vi "CliListBlocks.vi"(0 "ref in":u64, 11 "error in (no error)":errorcluster) -> (4 "ref out":u64, 6 "Result":i32, 8 "BlockList":T1, 15 "error out":errorcluster)   [LabVIEW 2019, in "Snap7.lvlib"]
uses:
  Snap7.lvlib
  windows/lv_snap7.dll
panel:
  in  "var BlockList":T1
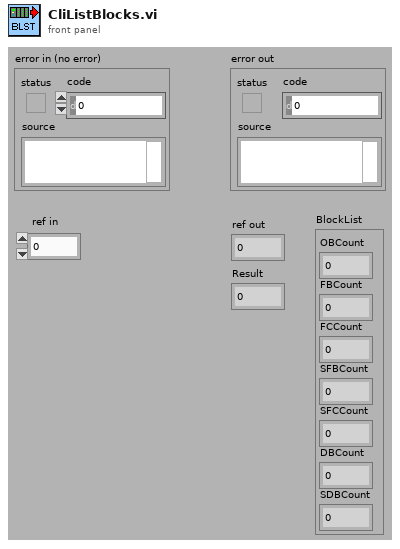
[diagram p1: front panel]
types:
  T1 = cluster{"OBCount":i32, "FBCount":i32, "FCCount":i32, "SFBCount":i32, "SFCCount":i32, "DBCount":i32, "SDBCount":i32}
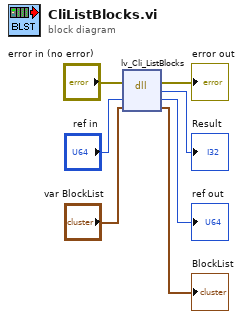
[diagram p0: block diagram]
diagram:
  n1 = dll-call lib="PTH2Xabs DSVNHLCEPStrunk性能试验台SourcesSnap7libwindowslv_snap7.dll" fn="lv_Cli_ListBlocks"(error in="error in (no error)", "Client"="ref in", "Cluster"="var BlockList") -> (error out=→"error out":errorcluster, "return type"=→"Result":i32, "Client"=→"ref out":u64, "Cluster"=→"BlockList":T1)  [unwired: 2 in, 1 out]
